vi "Headless Test.vi"() -> ()   [LabVIEW 2020, in "SquareBattle.lvlib"]
uses:
  SquareBattle.lvlib
  SB App/Team Status Data.ctl
  Team Stats.ctl
  Team State.ctl
  Squares/Demo/SquareTeam/MyTeam/MyTeam.lvclass
  C:/dev/illuminatedg/sol-squarebattle/SquareBattle/Team/Team.lvclass
  Squares/Clones/SquareTeam/MyTeam/MyTeam.lvclass
  Squares/DNatt/SquareTeam/MyTeam/MyTeam.lvclass
  Squares/Galaxy/SquareTeam/MyTeam/MyTeam.lvclass
  Squares/Rain/SquareTeam/MyTeam/MyTeam.lvclass
  3762ddda-4a42-4fb2-ad6b-13af8383e857.vi
  <vilib>/Utility/High Resolution Relative Seconds.vi
  Game/Game.lvclass
  <vilib>/ptbypt/NI_PtbyPt.lvlib
  SB App/SB App.lvlib
panel:
  out "Rate":dbl format="%#_2g"
  out "Team Stats":T1[](array[typedef])
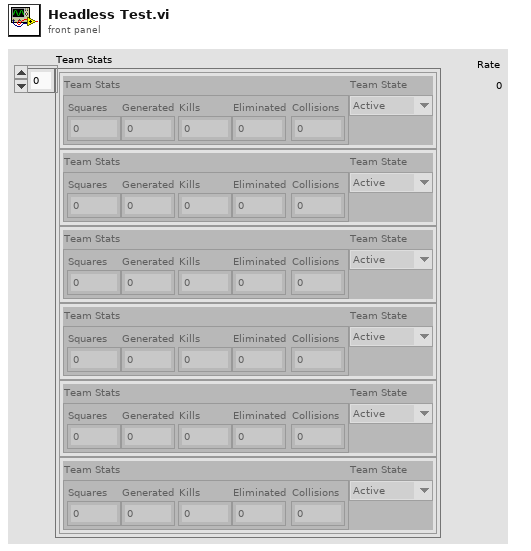
[diagram p1: front panel]
types:
  T1 = typedef "SB App.lvlib/Team Status Data.ctl" = cluster{"Team Stats":T2, "Team State":T3}
  T2 = typedef "SquareBattle.lvlib/Team Stats.ctl" = cluster{"Squares":i32, "Generated":i32, "Kills":i32, "Eliminated":i32, "Collisions":i32}
  T3 = typedef "SquareBattle.lvlib/Team State.ctl" = enum16{"Active", "Defeated", "Won"}
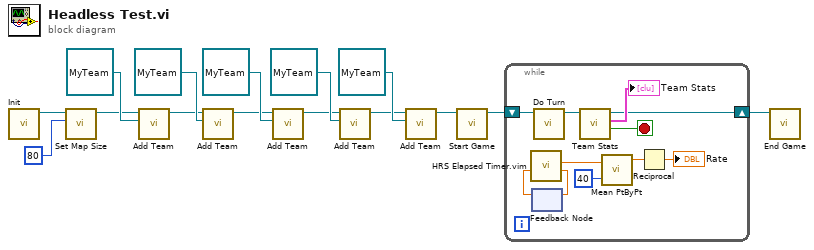
[diagram p0: block diagram]
diagram:
  n1 = call "Init.vi"() -> ("Game out"=w14:refnum<class "Game.lvclass">)  [unwired: 10 in, 1 out]
  n2 = call "Set Map Size.vi"("Map Size"=80, "Game in"=w14) -> ("Game out"=w12:refnum<class "Game.lvclass">)  [unwired: 8 in, 1 out]
  n3 = call "Add Team.vi"("Team Type"=refnum<class "MyTeam.lvclass"> refnum ("DemoTeam.lvlib:MyTeam.lvclass"), "Game in"=w12) -> ("Game out"=w4:refnum<class "Game.lvclass">)  [unwired: 7 in, 2 out]
  n4 = call "Add Team.vi"("Team Type"=refnum<class "MyTeam.lvclass"> refnum ("Clones.lvlib:MyTeam.lvclass"), "Game in"=w4) -> ("Game out"=w6:refnum<class "Game.lvclass">)  [unwired: 7 in, 2 out]
  n5 = call "Add Team.vi"("Team Type"=refnum<class "MyTeam.lvclass"> refnum ("DNattTeam.lvlib:MyTeam.lvclass"), "Game in"=w6) -> ("Game out"=w8:refnum<class "Game.lvclass">)  [unwired: 7 in, 2 out]
  n6 = call "Add Team.vi"("Team Type"=refnum<class "MyTeam.lvclass"> refnum ("Galaxy.lvlib:MyTeam.lvclass"), "Game in"=w8) -> ("Game out"=w10:refnum<class "Game.lvclass">)  [unwired: 7 in, 2 out]
  n7 = call "Add Team.vi"("Team Type"=refnum<class "MyTeam.lvclass"> refnum ("Rain.lvlib:MyTeam.lvclass"), "Game in"=w10) -> ("Game out"=w3:refnum<class "Game.lvclass">)  [unwired: 7 in, 2 out]
  n8 = call "Start Game.vi"("Game in"=w3) -> ("Game out"=w2:refnum<class "Game.lvclass">)  [unwired: 9 in, 1 out]
  n9 = while {
    shift-right: [w23] -> w1
    shift-left: w2 -> [w26]
    stop <- w22 stop-if-true
    n10 = feedback #1() -> (w21:dbl)  [unwired: 1 in]
    n11 = call "HRS Elapsed Timer.vim"("HRS In"=w21) -> ("HRS"=w20:dbl, "Elapsed"=w19:dbl)  [unwired: 7 in, 2 out]
    n12 = feedback-in #1(w20) -> ()
    n13 = call "Do Turn.vi"("Game in"=w26) -> ("Game out"=w25:refnum<class "Game.lvclass">)  [unwired: 10 in]
    n14 = call "Team Stats.vi"("Game in"=w25) -> ("Won?"=w22:bool, "Team Stats"=→"Team Stats":T1[], "Game out"=w23:refnum<class "Game.lvclass">)  [unwired: 7 in, 1 out]
    n15 = call <vilib>:"Mean PtByPt.vi"("x"=w19, "sample length"=40) -> ("mean"=w17:dbl)  [unwired: 2 in, 1 out]
    n16 = Reciprocal(x=w17) -> (1/x=→"Rate":dbl)
  }
  n17 = call "End Game.vi"("Game in"=w1) -> ()  [unwired: 9 in, 2 out]
